vi "Test Config Iface Default Path.vi"(8 "error in (no error)":errorcluster, 11 "Test Case In":refnum<class "Configuration Interface Test.lvclass">) -> (0 "error out":errorcluster, 3 "Test Case Out":refnum<class "Configuration Interface Test.lvclass">)   [LabVIEW 2020, in "Configuration Interface Test.lvclass"]
uses:
  Configuration Interface Test.lvclass
  C:/Program Files (x86)/National Instruments/LabVIEW 2020/vi.lib/Astemes/LUnit/Test Case.lvclass
  source/Framework/Configuration/Configuration.lvclass
  <vilib>/Astemes/LUnit/Test Case.lvclass/Test Case.ctl
  fbdc7d50-1976-4b35-96ba-616d9cd76990.vi
  <vilib>/Astemes/LUnit/Palette/Pass.vi
  <vilib>/Astemes/LUnit/Palette/Fail.vi
  <vilib>/Astemes/LUnit/Compare Variants.vi
  <vilib>/Astemes/LUnit/Describe Comparison.vi
  <vilib>/Astemes/LUnit/Set Assertion Type.vi
  <vilib>/Astemes/LUnit/Add test result.vi
  <vilib>/Astemes/LUnit/Variant to string.vi
  <vilib>/Astemes/LUnit/LUnit Record Assertion Result.vi
  <vilib>/Astemes/LUnit/LUnit Aggregate Assertion Results.vi
  <vilib>/Astemes/LUnit/Method Result/LUnit Merge Status.vi
  <vilib>/Astemes/LUnit/LUnit Concatenate result strings.vi
  <vilib>/Utility/Data Type/Get Type Information.vi
  <vilib>/Utility/LVClass/Get LV Class Name.vi
  Configuration Interface Test.lvclass/Configuration Interface Test.ctl
  <vilib>/Astemes/LUnit/Test Case.lvclass
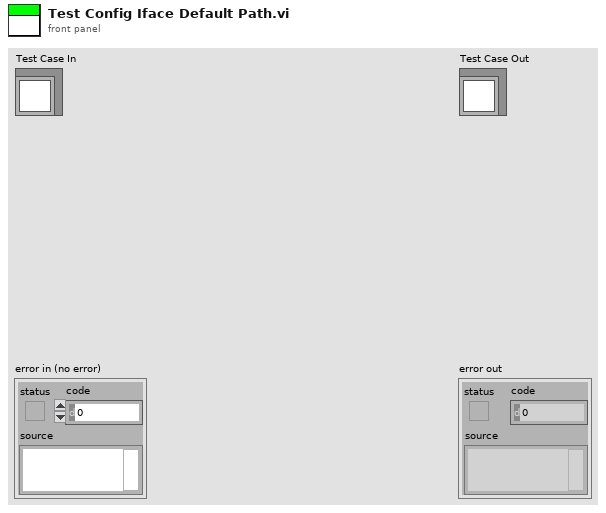
[diagram p1: front panel]
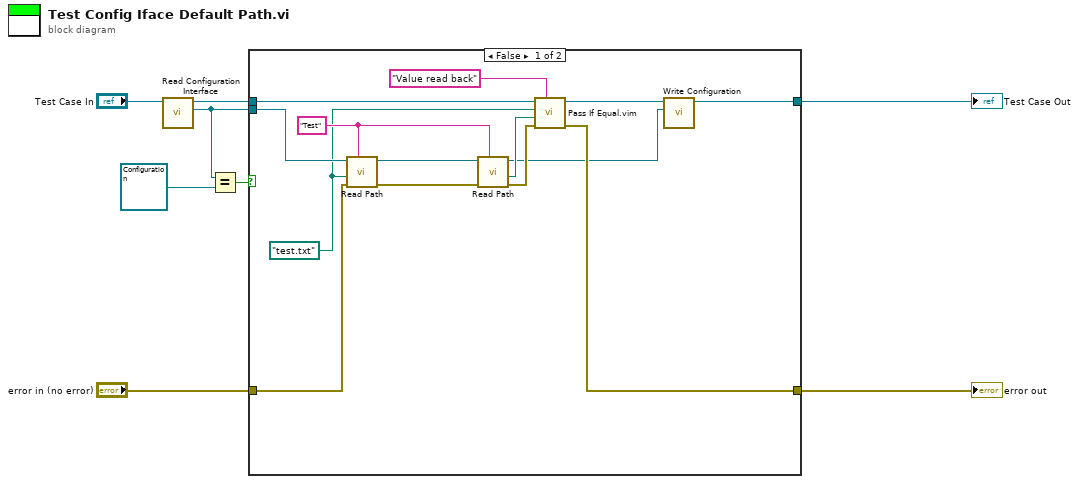
[diagram p0: block diagram]
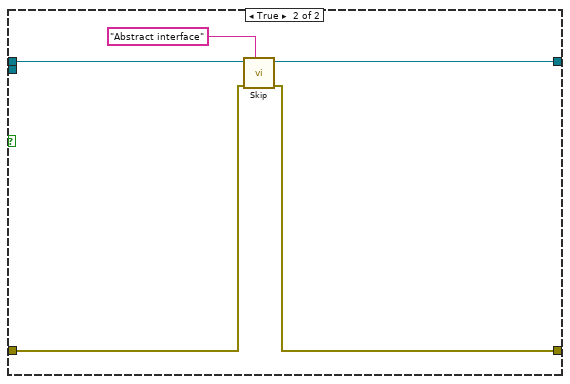
[diagram p2: hidden frame]
diagram:
  n1 = call "Read Configuration Interface.vi"("Configuration Interface Test In"="Test Case In") -> ("Configuration"=w3:refnum<class "Configuration.lvclass">, "Configuration Interface Test Out"=w6:refnum<class "Configuration Interface Test.lvclass">)  [unwired: 9 in]
  n2 = Equal?(x=w3, y=refnum<class "Configuration.lvclass"> refnum ("Configuration")) -> (x = y?=w1:bool)
  n3 = case shown="False" w1 {
    tunnel: [w19 w24] -> w7
    tunnel: w6 -> [w18 w27]
    tunnel: [w10 w26] -> w5
    tunnel: "error in (no error)" -> [w12 w25]
    tunnel: w3 -> [w15 _]
    frame False {
      w11 = path "test.txt"
      w20 = "Test" ("key")
      n4 = call-dynamic "Read Path.vi"("key"=w20, "error in (no error)"=w12, "default value"=w11, "Configuration In"=w15) -> ("error out"=w21:errorcluster, "Configuration Out"=w22:refnum<class "Configuration.lvclass">)  [unwired: 5 in, 1 out]
      n5 = call-dynamic "Read Path.vi"("key"=w20, "error in (no error)"=w21, "Configuration In"=w22) -> ("error out"=w16:errorcluster, "value"=w13:path, "Configuration Out"=w9:refnum<class "Configuration.lvclass">)  [unwired: 6 in]
      n6 = call "Pass If Equal.vim"("Description"="Value read back", "error in (no error)"=w16, "Actual"=w13, "Expected"=w11, "LUnit Test Case In"=w18) -> ("error out"=w19:errorcluster, "LUnit Test Case Out"=w17:refnum<class "Configuration Interface Test.lvclass">)  [unwired: 5 in]
      n7 = call "Write Configuration.vi"("Configuration"=w9, "Configuration Interface Test In"=w17) -> ("Configuration Interface Test Out"=w10:refnum<class "Configuration Interface Test.lvclass">)  [unwired: 8 in, 1 out]
    }
    frame True {
      n8 = call <vilib>:"Skip.vi"("Description"="Abstract interface", "error in (no error)"=w25, "LUnit Test Case In"=w27) -> ("error out"=w24:errorcluster, "LUnit Test Case Out"=w26:refnum<class "Configuration Interface Test.lvclass">)  [unwired: 7 in]
    }
  }
  "error out" <- w7
  "Test Case Out" <- w5
